vi "Init_Test.vi"(8 "error in (no error)":errorcluster caption="entrée d'erreur (pas d'erreur)", 11 "Get_Voltage en entrée":refnum<class "Init_SpectumAnalyser.lvclass">) -> (0 "error out":errorcluster caption="sortie d'erreur", 3 "Get_Voltage en sortie":refnum<class "Init_SpectumAnalyser.lvclass">)   [LabVIEW 2020, in "Library Test.lvlib" / "Init_SpectumAnalyser.lvclass"]
uses:
  Init_SpectumAnalyser.lvclass
  C:/Users/ngarcin/OneDrive - Altyor/Standard TB/Class/Test/Test (Default)/Test (Default).lvclass
  Commun VI/TypeDef/Commande Test/Commande Value Type.ctl
  Commun VI/TypeDef/Command Spectrum_Analyser/Parameter Spectrum_Analyser.ctl
  Spectrum Analyser/Class Spectrum Analyser (Default)/Class Spectrum Analyser (Default).lvclass
  JSON API/JSON Value/Set from JSON string.vi
  JSON API/Variant JSON/Variant to JSON.vi
  JSON API/JSON Value/Get Item by name array.vi
  Test_Wtih_Instr/Test_With_Inst.lvclass
  Instrument/Instrument (Default)/Class Instrument (Default).lvclass
  JSON API/JSON Value/JSON Value.lvclass
  Init_SpectumAnalyser.lvclass/Init_SpectumAnalyser.ctl
  Commun VI/Library Commun.lvlib
  JSON API/Variant JSON/Variant JSON.lvlib
  JSON API/Get Polymorphic/JSON GetSet.lvlib
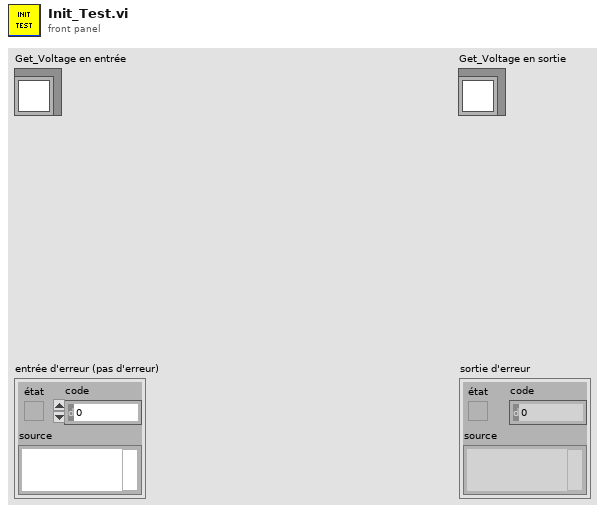
[diagram p1: front panel]
types:
  T1 = typedef "Library Commun.lvlib/Commande Value Type.ctl" = enum16{"None", "String", "Number", "Timestamp", "Boolean", "Array"}
  T2 = typedef "Parameter Spectrum_Analyser.ctl" = cluster{"Device @":string, "Class Spectrum Analyser":refnum<class "Class Spectrum Analyser (Default).lvclass">, "Center Freq (MHz)":dbl, "Freq Span (MHz)":dbl, "Ref Level (dBm)":dbl, "Threshold (dBm)":dbl, "TimeOut":i16}
  T3 = cluster{"Center Freq (MHz)":dbl, "Freq Span (MHz)":dbl, "Ref Level (dBm)":dbl, "Threshold (dBm)":dbl}
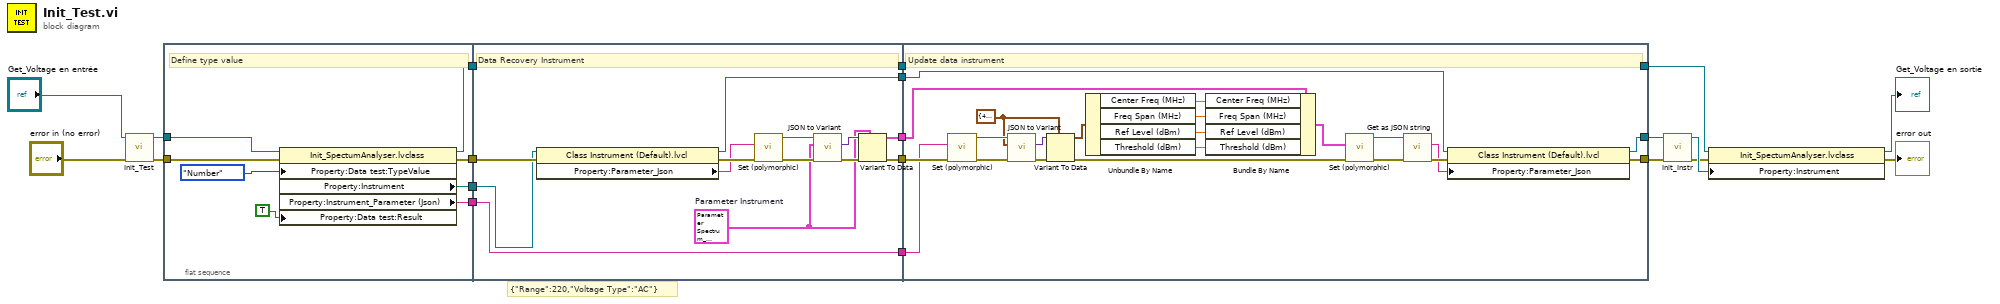
[diagram p0: block diagram]
diagram:
  # "{\"Range\":220,\"Voltage Type\":\"AC\"}"
  n1 = call-parent "Init_Test.vi"("error in (no error)"="error in (no error)", "Test_With_Inst en entrée"="Get_Voltage en entrée") -> ("error out"=w13:errorcluster, "Test_With_Inst en sortie"=w1:refnum<class "Init_SpectumAnalyser.lvclass">)  [unwired: 8 in]
  n2 = flat-sequence {
    tunnel: [w22] -> w15
    tunnel: [w25] -> w14
    tunnel: w1 -> [w28]
    tunnel: w13 -> [w27]
    tunnel: [w24] -> w11
    tunnel: [w23] -> w9
    tunnel: [w42] -> w18
    tunnel: [w32] -> w17
    tunnel: [w30] -> w16
    tunnel: w15 -> [w41]
    tunnel: w14 -> [w40]
    tunnel: [w31] -> w12
    tunnel: w11 -> [w31]
    tunnel: [w29] -> w10
    tunnel: w9 -> [w29]
    tunnel: w18 -> [w50]
    tunnel: w17 -> [w51]
    tunnel: w16 -> [w49]
    tunnel: [w47] -> w8
    tunnel: w12 -> [w48]
    tunnel: [w46] -> w7
    tunnel: w10 -> [w45]
    tunnel: [w45] -> w4
    frame #0 {
      # "Define type value"
      n3 = property class="Init_SpectumAnalyser.lvclass"(reference=w28, error in=w27, "Property:Data test:TypeValue"=Commande_Value_Type."Number" ("TypeValue"), "Property:Data test:Result"=TRUE ("Result")) -> (reference out=w23:refnum<class "Init_SpectumAnalyser.lvclass">, error out=w22:errorcluster, "Property:Instrument"=w25:refnum<class "Class Instrument (Default).lvclass">, "Property:Instrument_Parameter (Json)"=w24:string)
    }
    frame #1 {
      w33 = T2 {"Device @"="", "Class Spectrum Analyser"=refnum, "Center Freq (MHz)"=0.0, "Freq Span (MHz)"=0.0, "Ref Level (dBm)"=0.0, "Threshold (dBm)"=0.0, "TimeOut"=0}  # Parameter Instrument
      # "Data Recovery Instrument"
      n4 = property class="Class Instrument (Default).lvcl"(reference=w40, error in=w41) -> (reference out=w30:refnum<class "Class Instrument (Default).lvclass">, error out=w39:errorcluster, "Property:Parameter_Json"=w38:string)
      n5 = call-poly "Set (polymorphic).vi"("error in (no error)"=w39, "JSON stream"=w38) -> ("error out"=w36:errorcluster, "JSON Value out"=w34:refnum<class "JSON Value.lvclass">)  [unwired: 7 in, 1 out]
      n6 = call "JSON to Variant.vi"("error in (no error)"=w36, "Variant (Data Type)"=w33, "JSON Value"=w34) -> ("error out"=w35:errorcluster, "Variant out"=w37:variant)  [unwired: 7 in]
      n7 = Variant To Data(error in=w35, type=w33, Variant=w37) -> (data=w42:T2, error out=w32:errorcluster)
    }
    frame #2 {
      w44 = T3 {"Center Freq (MHz)"=433.0, "Freq Span (MHz)"=5.0, "Ref Level (dBm)"=10.0, "Threshold (dBm)"=-40.0} ("Cluster des données privées de classe")
      # "Update data instrument"
      n8 = call-poly "Set (polymorphic).vi"("error in (no error)"=w51, "JSON stream"=w48) -> ("error out"=w53:errorcluster, "JSON Value out"=w55:refnum<class "JSON Value.lvclass">)  [unwired: 7 in, 1 out]
      n9 = call "JSON to Variant.vi"("error in (no error)"=w53, "Variant (Data Type)"=w44, "JSON Value"=w55) -> ("error out"=w54:errorcluster, "Variant out"=w52:variant)  [unwired: 7 in]
      n10 = Variant To Data(error in=w54, type=w44, Variant=w52) -> (data=w56:T3, error out=w62:errorcluster)
      n11 = Unbundle By Name(w56) -> ("Center Freq (MHz)"=w57:dbl, "Freq Span (MHz)"=w58:dbl, "Ref Level (dBm)"=w59:dbl, "Threshold (dBm)"=w43:dbl)
      n12 = Bundle By Name(cluster=w50, "Center Freq (MHz)"=w57, "Freq Span (MHz)"=w58, "Ref Level (dBm)"=w59, "Threshold (dBm)"=w43) -> (w63:T2)
      n13 = call-poly "Set (polymorphic).vi"("error in (no error)"=w62, "Variant"=w63) -> ("error out"=w60:errorcluster, "JSON Value out"=w61:refnum<class "JSON Value.lvclass">)  [unwired: 8 in]
      n14 = call "Get as JSON string.vi"("error in (no error)"=w60, "JSON Value in"=w61) -> ("error out"=w65:errorcluster, "<JSON>"=w64:string)  [unwired: 8 in]
      n15 = property class="Class Instrument (Default).lvcl"(reference=w49, error in=w65, "Property:Parameter_Json"=w64) -> (reference out=w46:refnum<class "Class Instrument (Default).lvclass">, error out=w47:errorcluster)
    }
  }
  n16 = call-dynamic "Init_Instr.vi"("error in (no error)"=w8, "Class Instrument (Default) en entrée"=w7) -> ("error out"=w3:errorcluster, "Class Instrument (Default) en sortie"=w6:refnum<class "Class Instrument (Default).lvclass">)  [unwired: 8 in]
  n17 = property class="Init_SpectumAnalyser.lvclass"(reference=w4, error in=w3, "Property:Instrument"=w6) -> (reference out=→"Get_Voltage en sortie":refnum<class "Init_SpectumAnalyser.lvclass">, error out=→"error out":errorcluster)
